vi "Set DIO Port AB Bit Status.vi"(4 "error in (no error)":errorcluster, 6 "DIO Port status":T1={"Port A bit-0 at logic level"=TRUE, "Port A bit-1 at logic level"=TRUE, "Port A bit-2 at logic level "=TRUE, "Port A bit-3 at logic level"=TRUE, "Port A bit-4 at logic level"=TRUE, "Port A bit-5 at logic level "=TRUE, "Port A bit-6 at logic level "=TRUE, "Port A bit-7 at logic level "=TRUE, "Port B bit-0 at logic level"=TRUE, "Port B bit-1 at logic level"=TRUE, "Port B bit-2 at logic level "=TRUE, "Port B bit-3 at logic level"=TRUE, "Port B bit-4 at logic level"=TRUE, "Port B bit-5 at logic level "=TRUE, "Port B bit-6 at logic level "=TRUE, "Port B bit-7 at logic level "=TRUE}, 7 "VISA resource name":refnum<visa-resource-name>) -> (0 "error out":errorcluster, 3 "VISA resource name out":refnum<visa-resource-name>)   [LabVIEW 2012, in "Newport ESP301.lvlib"]
doc: "Gets all digital I/O port A,B and C logic level.\nThis command is used to either set all digital I/O (DIO) port A, B, and C logic level or read its present status. Bits 0-7 correspond to port A, and bits 8-15 to port B. Each 8-bit port can be set as either input or output with the BO command.\nA DIO within a port configured as an input can only report its present HIGH or LOW logic level. Whereas a DIO bit within a port configured as an output can set(1) or clear(0) the corresponding DIO hardware to HIGH or LOW logic level.\nReading the status of a port configured as output returns its present output status.\n<B>NOTE</B>: All direction bits are automatically zeroed, or cleared, after a system reset. Therefore all DIO ports default to input by default.\n<B>NOTE</B>: Each DIO bit has a pulled-up resistor to +5V. Therefore, all bits will be at HIGH logic level if not connected to external circuit and configured as input."
uses:
  Newport ESP301.lvlib
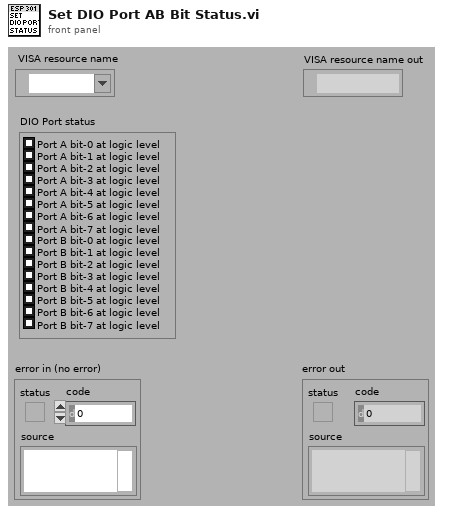
[diagram p1: front panel]
types:
  T1 = cluster{"Port A bit-0 at logic level":bool, "Port A bit-1 at logic level":bool, "Port A bit-2 at logic level ":bool, "Port A bit-3 at logic level":bool, "Port A bit-4 at logic level":bool, "Port A bit-5 at logic level ":bool, "Port A bit-6 at logic level ":bool, "Port A bit-7 at logic level ":bool, "Port B bit-0 at logic level":bool, "Port B bit-1 at logic level":bool, "Port B bit-2 at logic level ":bool, "Port B bit-3 at logic level":bool, "Port B bit-4 at logic level":bool, "Port B bit-5 at logic level ":bool, "Port B bit-6 at logic level ":bool, "Port B bit-7 at logic level ":bool}
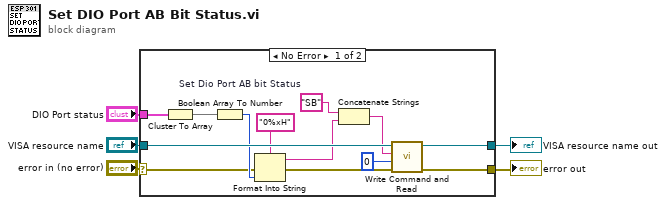
[diagram p0: block diagram]
diagram:
  n1 = case shown="No Error" "error in (no error)" {
    selector: "error in (no error)" -> [w10 w20]
    tunnel: [w17 w20] -> w5
    tunnel: "VISA resource name" -> [w18 w19]
    tunnel: [w16 w19] -> w4
    tunnel: "DIO Port status" -> [w7 _]
    frame No Error {
      w15 = "SB"  # Set Dio Port AB bit Status
      n2 = Cluster To Array(cluster=w7) -> (array=w12:bool[])
      n3 = Boolean Array To Number(Boolean array=w12) -> (number=w11:u32)
      n4 = Format Into String(format string="0%xH" ("chaîne de format"), error in=w10, w11) -> (resulting string=w8:string, error out=w9:errorcluster)  [unwired: 1 in]
      n5 = Concatenate Strings(w15, w8) -> (w14:string)
      n6 = call "Write Command and Read.vi"("error in (no error)"=w9, "Bytes to read (100)"=u32 0, "Command"=w14, "VISA resource name"=w18) -> ("error out"=w17:errorcluster, "VISA resource name out"=w16:refnum<visa-resource-name>)  [unwired: 1 in, 3 out]
    }
    frame Error {
    }
  }
  "error out" <- w5
  "VISA resource name out" <- w4
